vi "Read Temperature.vi"(8 "error in (no error)":errorcluster, 11 "thermal sensor":refnum<class "Thermal Sensor.lvclass">) -> (0 "error out":errorcluster, 2 "temperature":dbl[unit]=273.15)   [LabVIEW 2023, in "Thermal Sensor.lvclass"]
uses:
  Thermal Sensor.lvclass
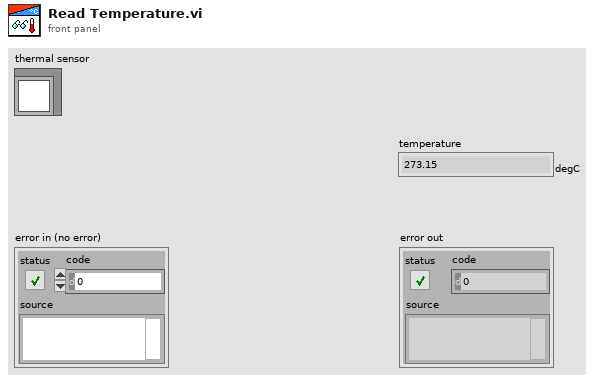
[diagram p1: front panel]
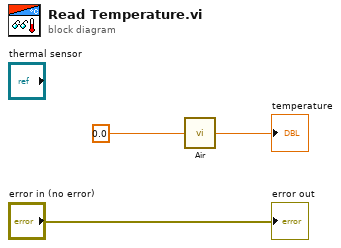
[diagram p0: block diagram]
diagram:
  n1 = call "Air.vi"("temperature adjustment"=dbl[unit] 0.0 ("Temperature")) -> ("new air temperature"=→"temperature":dbl[unit])
  "error out" <- "error in (no error)"
